vi "Init.vi"(8 "error in (no error)":errorcluster, 11 "Controller Map":T1) -> (0 "error out":errorcluster, 3 "PathRegex Router out":refnum<class "PathRegex Router.lvclass">)   [LabVIEW 2020, in "HTTP Server.lvlib" / "PathRegex Router.lvclass"]
uses:
  PathRegex Router.lvclass
  Controller/Controller.lvclass
  Priority.ctl
  HTTP Server.lvlib
  Controller Map.ctl
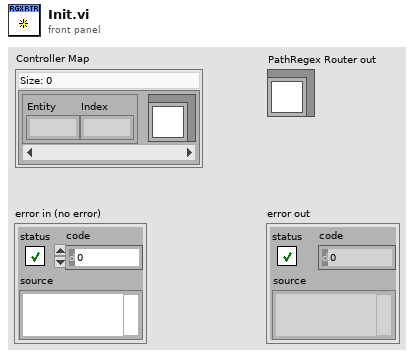
[diagram p1: front panel]
types:
  T1 = typedef "HTTP Server.lvlib/Controller Map.ctl" = map{T2, refnum<class "Controller.lvclass">}
  T2 = typedef "HTTP Server.lvlib/Priority.ctl" = cluster{"Entity":u16, "Index":u16}
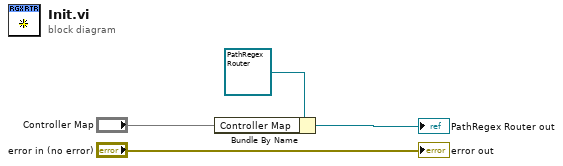
[diagram p0: block diagram]
diagram:
  n1 = Bundle By Name(cluster=refnum<class "PathRegex Router.lvclass"> refnum ("PathRegex Router out"), "Controller Map"="Controller Map") -> (→"PathRegex Router out":refnum<class "PathRegex Router.lvclass">)
  "error out" <- "error in (no error)"
